vi "BB_TestCOM.vi"() -> ()   [LabVIEW 2012]
uses:
  SubVIs/LVPresent_Globals.vi
  <userlib>/BotSpeak/VIs/SubVIs/BotSpeak_Globals.vi
  BotSpeakSubs/BotspeakSettingsUsed.vi
panel:
  in  "Combo Box":string(combo)
  out "Status":string
  in  "Test Button":bool
  in  "Hardware":u16(ring)=2 items=["Arduino Uno", "BeagleBone Serial", "BeagleBone", "Console Only", "EV3", "Launchpad", "PICAXE 80M", "Raspberry Pi", "Thymio"]
  out "Connect?":bool
  # "Test BotSpeak\n\nThe next step is to test it out.  Choose your hardware and port (if you have not plugged your BeagleBone in yet, plug it in and select BeagleBone). You should get a green square after a few seconds if you are connected. Click the next arrow once you are connected."
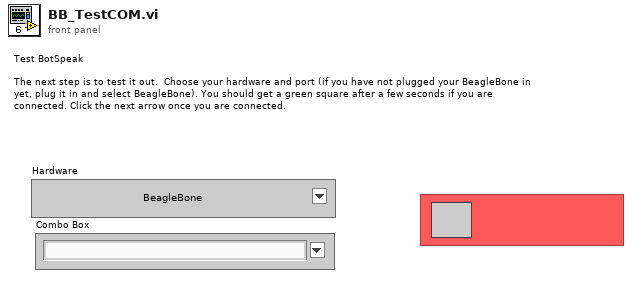
[diagram p1: front panel]
types:
  T1 = typedef "BotSpeak.HardwareSpecs.ctl" = cluster{"Hardware Name":string, "Hardware URL":string, "ComType":enum16{"Undefined", "Serial", "TCPIP", "Console", "EV3"}, "TCP Port":i32, "DefaultAddress":string, "Retries":i32, "Translate":enum16{"None", "Tiny", "URAPI"}, "MaxScriptSize":i32, "MaxVarNumber":i32, "StartupWait":i32, "Patience":i32, "Startup Patience":i32, "Hardware Help":string, "Com Protocol":string, "Translator":cluster{"BotSpeak CMD":string, "CMD out":string}[], "Init Code":string, "Variable Format":enum16{"INT", "FLOAT", "FIXED"}}
  T2 = typedef "BotSpeak_Control.ctl" = cluster{"Address":string, "Reply EOF":string, "Hardware":string, "Retries":i8, "Timeout":i32}
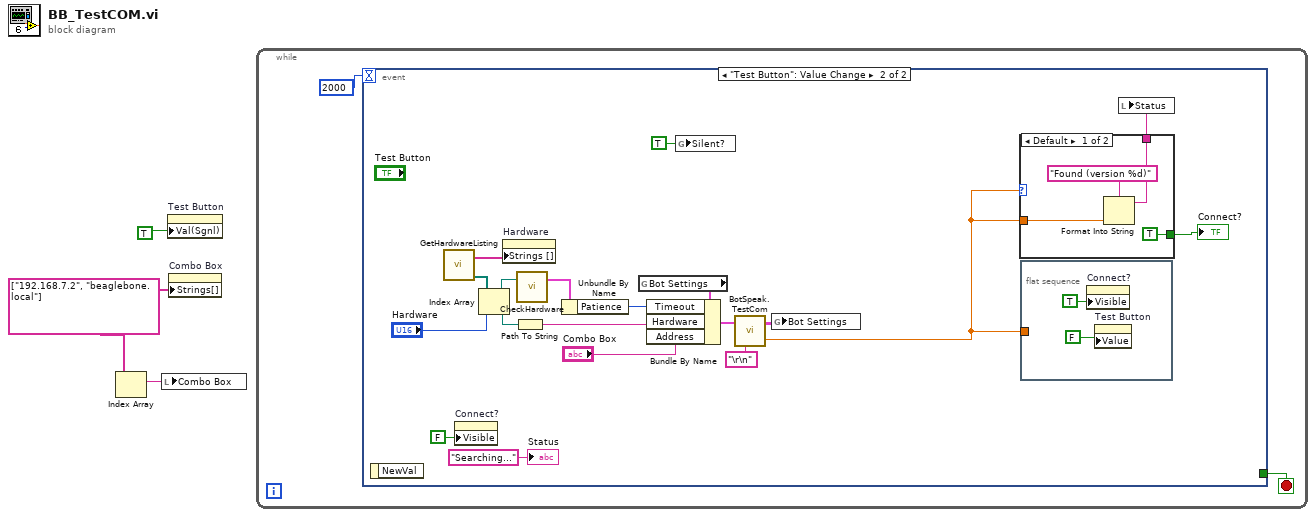
[diagram p0: block diagram]
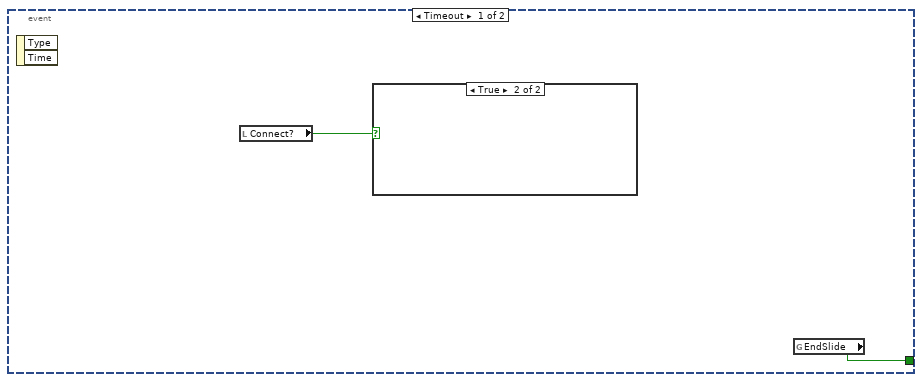
[diagram p2: hidden frame]
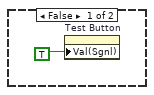
[diagram p3: hidden frame]
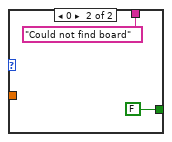
[diagram p4: hidden frame]
diagram:
  w2 = string[] ["192.168.7.2", "beaglebone.local"] ("Strings []")
  n1 = Index Array(array=w2) -> (element=w1:string)  [unwired: 1 in]
  n2 = local write "Combo Box"(w1) -> ()
  n3 = property on="Test Button" class="Bool (strict)"("Val(Sgnl)"=TRUE) -> ()  [unwired: 2 in, 2 out]
  n4 = property on="Combo Box" class="CmbBox"("Strings[]"=w2) -> ()  [unwired: 2 in, 2 out]
  n5 = while {
    stop <- w5 stop-if-true
    n6 = event shown="[1] \"Test Button\": Value Change" {
      selector: _ -> [_ _]
      dyn-events: _ -> [_ _]
      timeout: 2000 -> [_ _]
      tunnel: [w7 _] -> w5
      event Timeout {
        n7 = event-data() -> ()  [unwired: 1 in, 2 out]
        n8 = local read "Connect?"() -> (w6:bool)
        n9 = case shown="True" w6 {
          frame False {
            n10 = property on="Test Button" class="Bool (strict)"("Val(Sgnl)"=TRUE) -> ()  [unwired: 2 in, 2 out]
          }
          frame True {
          }
        }
        n11 = global read "LVPresent_Globals.vi" "EndSlide"() -> (w7:bool)
      }
      event "Test Button": Value Change {
        n12 = event-data() -> ()  [unwired: 1 in, 1 out]
        n13 = call <userlib>:"GetHardwareListing.vi"() -> ("Devices"=w21:path[], "Array"=w26:string[])  [unwired: 2 in]
        n14 = property on="Connect?" class="Bool (strict)"("Visible"=FALSE) -> ()  [unwired: 2 in, 2 out]
        n15 = Index Array(array=w21, index="Hardware") -> (element=w20:path)
        n16 = property on="Hardware" class="Ring (strict)"("Strings []"=w26) -> ()  [unwired: 2 in, 2 out]
        n17 = Path To String(path=w20) -> (string=w24:string)
        n18 = call <userlib>:"CheckHardware.vi"("Hardware"=w20) -> ("HardwareSpecs"=w17:T1)  [unwired: 2 in]
        n19 = Unbundle By Name(w17) -> ("Patience"=w23:i32)
        n20 = global read "BotspeakSettingsUsed.vi" "Bot Settings"() -> (w19:T2)
        n21 = Bundle By Name(cluster=w19, "Timeout"=w23, "Hardware"=w24, "Address"="Combo Box") -> (w22:T2)
        n22 = global write "BotSpeak_Globals.vi" "Silent?"(TRUE ("Silent?")) -> ()
        n23 = call <userlib>:"BotSpeak.TestCom.vi"("Termination"="\r\n", "Bot Settings"=w22) -> ("firmware"=w14:dbl, "Bot Settings out"=w16:T2)
        n24 = global write "BotspeakSettingsUsed.vi" "Bot Settings"(w16) -> ()
        n25 = case shown="Default" w14 {
          tunnel: w14 -> [w29 _]
          tunnel: [w28 "Could not find board"] -> w13
          tunnel: [TRUE FALSE] -> w12
          frame Default {
            n26 = Format Into String(format string="Found (version %d)" ("Status"), w29) -> (resulting string=w28:string)  [unwired: 2 in, 1 out]
          }
          frame 0 {
          }
        }
        "Connect?" <- w12
        n27 = flat-sequence {
          tunnel: w14 -> [_]
          frame #0 {
            n28 = property on="Connect?" class="Bool (strict)"("Visible"=TRUE) -> ()  [unwired: 2 in, 2 out]
            n29 = property on="Test Button" class="Bool (strict)"("Value"=FALSE) -> ()  [unwired: 2 in, 2 out]
          }
        }
        n30 = local write "Status"(w13) -> ()
        "Status" <- "Searching..." ("Status")
      }
    }
  }
